vi "ChangeSessionV2.vi"(1 "error in (no error)":errorcluster, 2 "Session":string="D:\\STM Data\\082016\\test") -> (0 "error out":errorcluster)   [LabVIEW 2014]
panel:
  in  "AutoItX3Lib.IAutoItX3":refnum<k7>
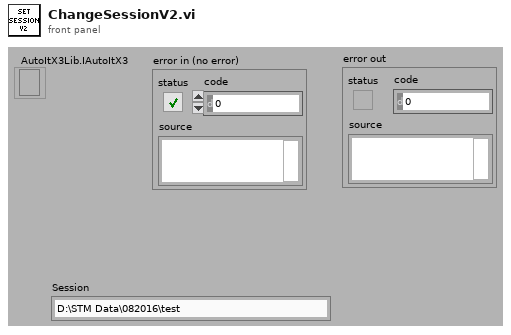
[diagram p1: front panel]
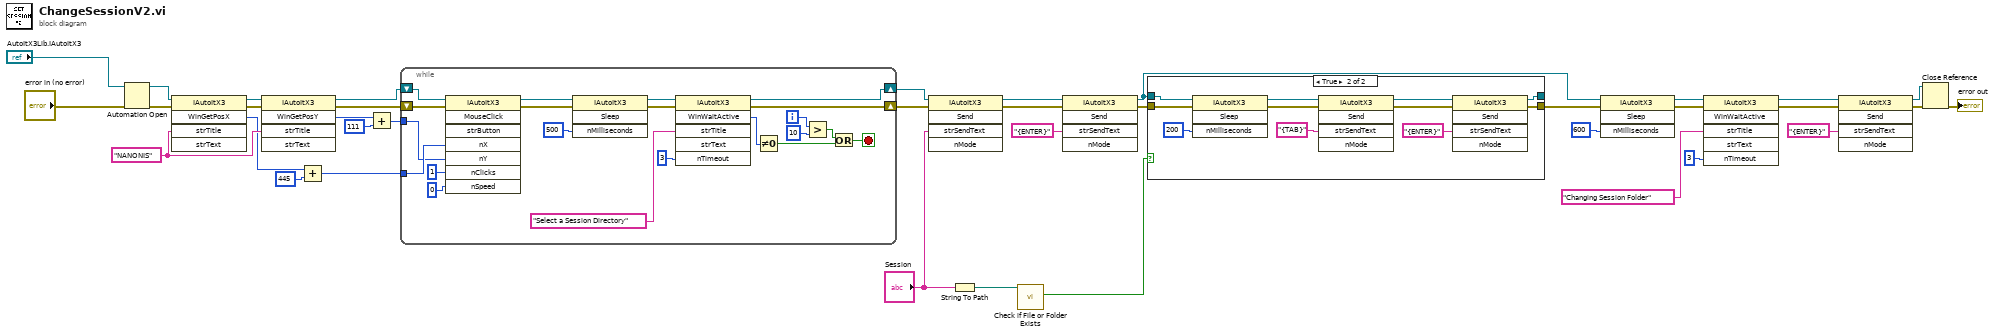
[diagram p0: block diagram]
diagram:
  w21 = "NANONIS" ("strTitle")
  n1 = Automation Open(error in (no error)="error in (no error)", Automation Refnum="AutoItX3Lib.IAutoItX3") -> (Automation Refnum=w28:refnum<k7>, error out=w29:errorcluster)  [unwired: 2 in]
  n2 = invoke class="IAutoItX3" method="WinGetPosX"(reference=w28, error in=w29, "strTitle"=w21) -> (reference out=w19:refnum<k7>, error out=w20:errorcluster, "WinGetPosX"=w17:i32)  [unwired: 2 in, 2 out]
  n3 = invoke class="IAutoItX3" method="WinGetPosY"(reference=w19, error in=w20, "strTitle"=w21) -> (reference out=w36:refnum<k7>, error out=w35:errorcluster, "WinGetPosY"=w18:i32)  [unwired: 2 in, 2 out]
  n4 = Add(x=w17, y=445) -> (x+y=w16:i32)
  n5 = Add(x=w18, y=111) -> (x+y=w14:i32)
  n6 = while {
    tunnel: w16 -> [w56]
    tunnel: w14 -> [w55]
    shift-right: [w47] -> w5
    shift-left: w36 -> [w58]
    shift-right: [w48] -> w6
    shift-left: w35 -> [w57]
    i -> [w41]
    stop <- w40 stop-if-true
    n7 = invoke class="IAutoItX3" method="MouseClick"(reference=w58, error in=w57, "nX"=w56, "nY"=w55, "nClicks"=1, "nSpeed"=0) -> (reference out=w54:refnum<k7>, error out=w53:errorcluster)  [unwired: 2 in, 6 out]
    n8 = invoke class="IAutoItX3" method="Sleep"(reference=w54, error in=w53, "nMilliseconds"=500) -> (reference out=w49:refnum<k7>, error out=w46:errorcluster)  [unwired: 1 in, 2 out]
    n9 = invoke class="IAutoItX3" method="WinWaitActive"(reference=w49, error in=w46, "strTitle"="Select a Session Directory", "nTimeout"=3) -> (reference out=w47:refnum<k7>, error out=w48:errorcluster, "WinWaitActive"=w43:i32)  [unwired: 2 in, 3 out]
    n10 = Not Equal To 0?(x=w43) -> (x != 0?=w42:bool)
    n11 = Greater?(x=w41, y=10) -> (0:w39:bool)
    n12 = Or(x=w39, y=w42) -> (x .or. y?=w40:bool)
  }
  n13 = invoke class="IAutoItX3" method="Send"(reference=w5, error in=w6, "strSendText"="Session") -> (reference out=w26:refnum<k7>, error out=w25:errorcluster)  [unwired: 2 in, 3 out]
  n14 = String To Path(string="Session") -> (path=w11:path)
  n15 = call <vilib>:"Check if File or Folder Exists.vi"("path"=w11) -> ("file or folder exists?"=w10:bool)  [unwired: 8 in, 2 out]
  n16 = invoke class="IAutoItX3" method="Send"(reference=w26, error in=w25, "strSendText"="{ENTER}") -> (reference out=w9:refnum<k7>, error out=w8:errorcluster)  [unwired: 2 in, 3 out]
  n17 = case shown="True" w10 {
    tunnel: w9 -> [w60 w62]
    tunnel: [w60 w70] -> _
    tunnel: w8 -> [w59 w63]
    tunnel: [w59 w69] -> w7
    frame False {
    }
    frame True {
      n18 = invoke class="IAutoItX3" method="Sleep"(reference=w62, error in=w63, "nMilliseconds"=200) -> (reference out=w61:refnum<k7>, error out=w64:errorcluster)  [unwired: 1 in, 2 out]
      n19 = invoke class="IAutoItX3" method="Send"(reference=w61, error in=w64, "strSendText"="{TAB}") -> (reference out=w71:refnum<k7>, error out=w68:errorcluster)  [unwired: 2 in, 3 out]
      n20 = invoke class="IAutoItX3" method="Send"(reference=w71, error in=w68, "strSendText"="{ENTER}") -> (reference out=w70:refnum<k7>, error out=w69:errorcluster)  [unwired: 2 in, 3 out]
    }
  }
  n21 = invoke class="IAutoItX3" method="Sleep"(reference=w9, error in=w7, "nMilliseconds"=600) -> (reference out=w24:refnum<k7>, error out=w23:errorcluster)  [unwired: 1 in, 2 out]
  n22 = invoke class="IAutoItX3" method="WinWaitActive"(reference=w24, error in=w23, "strTitle"="Changing Session Folder", "nTimeout"=3) -> (reference out=w32:refnum<k7>, error out=w31:errorcluster)  [unwired: 2 in, 4 out]
  n23 = invoke class="IAutoItX3" method="Send"(reference=w32, error in=w31, "strSendText"="{ENTER}" ("strTitle")) -> (reference out=w4:refnum<k7>, error out=w3:errorcluster)  [unwired: 2 in, 3 out]
  n24 = Close Reference(reference=w4, error in (no error)=w3) -> (error out=→"error out":errorcluster)
